vi "Found tp information.vi"(11 "TP DATA":string) -> (0 "H/W Config File":string, 1 "Comments":string, 2 "Author":string, 3 "UUT Model":string, 4 "TP Information(array)":string[](array[string]), 5 "Board Col":string, 6 "HW CH Number":string, 7 "Board Row":string)   [LabVIEW 2018]
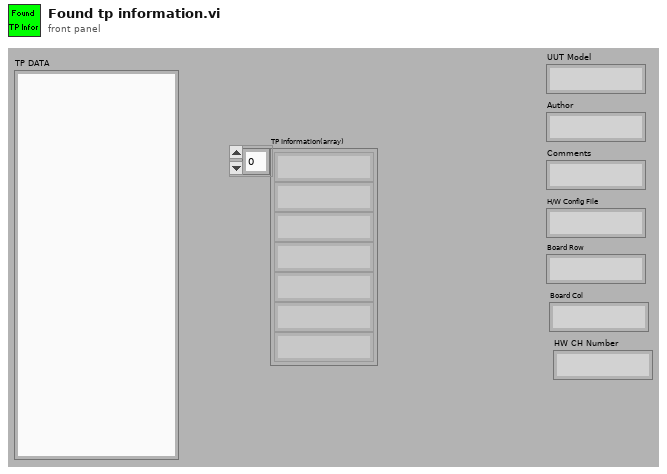
[diagram p1: front panel]
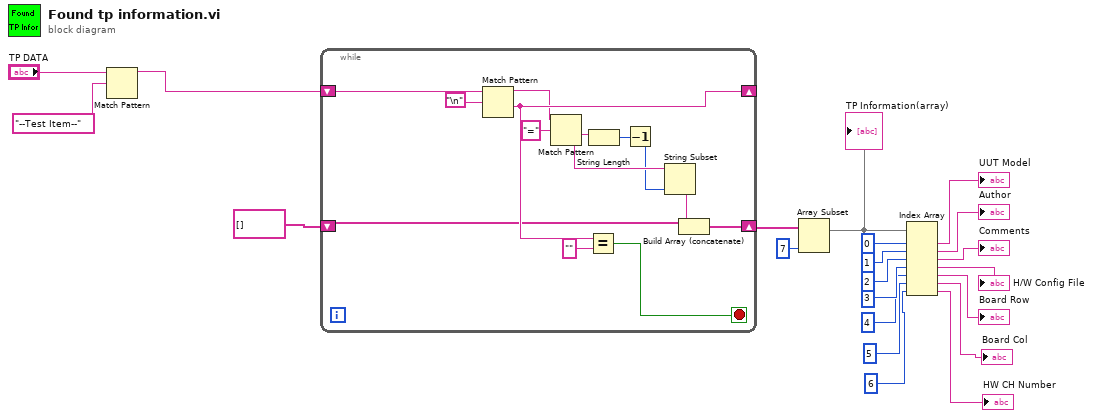
[diagram p0: block diagram]
diagram:
  n1 = Match Pattern(string="TP DATA", regular expression="--Test Item--") -> (before substring=w20:string)  [unwired: 4 out]
  n2 = while {
    shift-right: [w30] -> _
    shift-left: w20 -> [w34]
    shift-right: [w29] -> w17
    shift-left: string[] [] -> [w28]
    stop <- w31 stop-if-true
    n3 = Match Pattern(string=w34, regular expression="\n") -> (before substring=w26:string, after substring=w30:string)  [unwired: 3 out]
    n4 = Match Pattern(string=w26, regular expression="=") -> (after substring=w24:string)  [unwired: 4 out]
    n5 = Equal?(x=w30, y="") -> (x = y?=w31:bool)
    n6 = String Length(string=w24) -> (length=w25:i32)
    n7 = Decrement(x=w25) -> (x-1=w23:i32)
    n8 = String Subset(string=w24, length (rest)=w23) -> (substring=w22:string)  [unwired: 1 out]
    n9 = Build Array (concatenate)(w28, w22) -> (w29:string[])
  }
  n10 = Array Subset(array=w17, length=7) -> (w15:string[])  [unwired: 1 in]
  "TP Information(array)" <- w15
  n11 = Index Array(array=w15, index #1=0, index #2=1, index #3=2, index #4=3, index #5=4, index #6=5, index #7=6) -> (element #1=→"UUT Model":string, element #2=→"Author":string, element #3=→"Comments":string, element #4=→"H/W Config File":string, element #5=→"Board Row":string, element #6=→"Board Col":string, element #7=→"HW CH Number":string)
